vi "S4ACS.vi"() -> ()   [LabVIEW 2018]
uses:
  SPARC4_Channel/SPARC4_Channel.lvclass
  C:/Users/Denis/Desktop/S4ACS/S4ACS/Channel/Channel.lvclass
  Channel/Channel.lvclass/Channel.ctl
  Server/Server.lvclass/Server.ctl
  SPARC4_Channel/SPARC4_Channel.lvclass/SPARC4_Channel.ctl
  Sim_CCD/Sim_CCD.lvclass/Sim_CCD.ctl
  Sim_Ixon_Ultra/Sim_Ixon_Ultra.lvclass
  C:/Users/Denis/Desktop/S4ACS/S4ACS/Sim_CCD/Sim_CCD.lvclass
  <vilib>/Utility/error.llb/Error Cluster From Error Code.vi
  Sim_CCD/Sim_CCD.lvclass
  RxTx/RxTx.lvclass
  <vilib>/ErrorRing/Error Ring.xnode
  Channel/Channel.lvclass
  Server/Server.lvclass
panel:
  in  "generate error":bool
  out "error out":errorcluster
  in  "Tab Control":T1(tab)
  in  "Configuration to initialize ACS":T2={"image path"=path "C:/images/today", "channel"=1, "s4acs mode"=0, "log file path"=path "C:/sparc4/log/s4acs1", "min. log level"=0} {"min. log level" items=["STATUS", "DEBBUG", "INFO", "WARNING", "ERROR", "CRITICAL"]; "s4acs mode" items=["simulated", "real"]; "channel" min=1 max=4}
  out "S4GUI":bool
  out "S4ICS":bool
  out "TCS":bool
  out "Weather Station":bool
  out "Tel. focuser":bool
  out "wait expose cmd":bool
  in  "Stop Button":bool
  in  "software version":string="v1.56.0"
  out "ccd on/off":bool
  in  "use config file":bool=TRUE
  out "execution error":bool
  out "Numeric 2":i32
  out "Error Message":string
  out "Acquiring 2":bool
  out "Numeric":i32
  out "Code error message":string
  out "#cycles":u32
  out "cycles done":u16
  out "#seqs":u32
  out "seqs done":u16
  out "last update":string
  out "s4gui message":string
  out "last image":string
  out "frames done":u16
  out "ccd status":string
  out "temp (ºC)":i16
  out "temperature status":string
  out "exptime (s)":dbl
  out "serial number":u16
  out "Acquiring":bool
  out "#frames":u32
  in  "video mode":bool
  in  "reset axis":bool
  in  "contrast":dbl(slide)=1.0 scale=0.0..1.0
  in  "counts level":dbl(slide)=15.0 scale=0.0..5.0
  out "Intensity Graph":u16[][](graph)
  out "Header CCD Config":T3={"EM_GAIN"=2, "FRAME_TRANSFER"=TRUE, "SHUTTER_OPENING_TIME"=50, "SHUTTER_CLOSING_TIME"=50, "VBIN"=1, "INITIAL_LINE"=1, "INITIAL_COLUMN"=1, "FINAL_LINE"=1024, "FINAL_COLUMN"=1024, "HBIN"=1, "AD_CHANNEL"=0, "EM_MODE"=1, "PREAMP"=0, "SHUTTER_TTL"=0, "SHUTTER_MODE"=2, "ACQUISITION_MODE"=3, "TRIGGER_MODE"=0, "VERTICAL_CLOCK_VOLTAGE"=0, "VERTICAL_SHIFT_SPEED"=3, "READ_MODE"=4, "Last update"=timestamp(0 s since 1904-01-01), "READOUT_RATE"=""} {"READ_MODE" items=["Full Vertical Binning", "Multi-track", "Random-track", "Single-track", "Image"]; "VERTICAL_SHIFT_SPEED" items=["0.6", "1.13", "2.2", "4.33"]; "VERTICAL_CLOCK_VOLTAGE" items=["0", "+1", "+2", "+3", "+4"]; "TRIGGER_MODE" items=["Internal", "External", "N/A", "N/A_1", "N/A_2", "N/A_3", "External Start"]; "ACQUISITION_MODE" items=["Reserved", "Single", "Accumulate", "Kinetic"]; "SHUTTER_MODE" items=["Auto", "Open", "Closed"]; "SHUTTER_TTL" items=["TTL Low", "TTL High"]; "PREAMP" items=["Gain 1", "Gain 2"]; "EM_MODE" items=["Electron Multiplying", "Conventional"]}
  out "ACS status":string
  out "S4GUI":string
  out "S4ICS":string
  out "TCS":string
  out "Focuser":string
  out "Weather station":string
  out "SET erros":errorcluster
  out "Execution errors":errorcluster
  out "WRITE SETUP errors":errorcluster[](array[cluster])
  # "SPARC4 Acquisiton Control System (S4ACS)"
  # "Init communication"
  # "CCD status"
  # "ccd op. mode error"
  # "execution error"
  # "x1000"
  # "Camera configuration"
  # "Communication with the sub-systems of the observatory"
  # "Errors found during the exection of S4ACS"
  # "- Errors related to the WRITE SETUP command:"
  # "- Errors related to the SET command:"
  # "- Execution errors:"
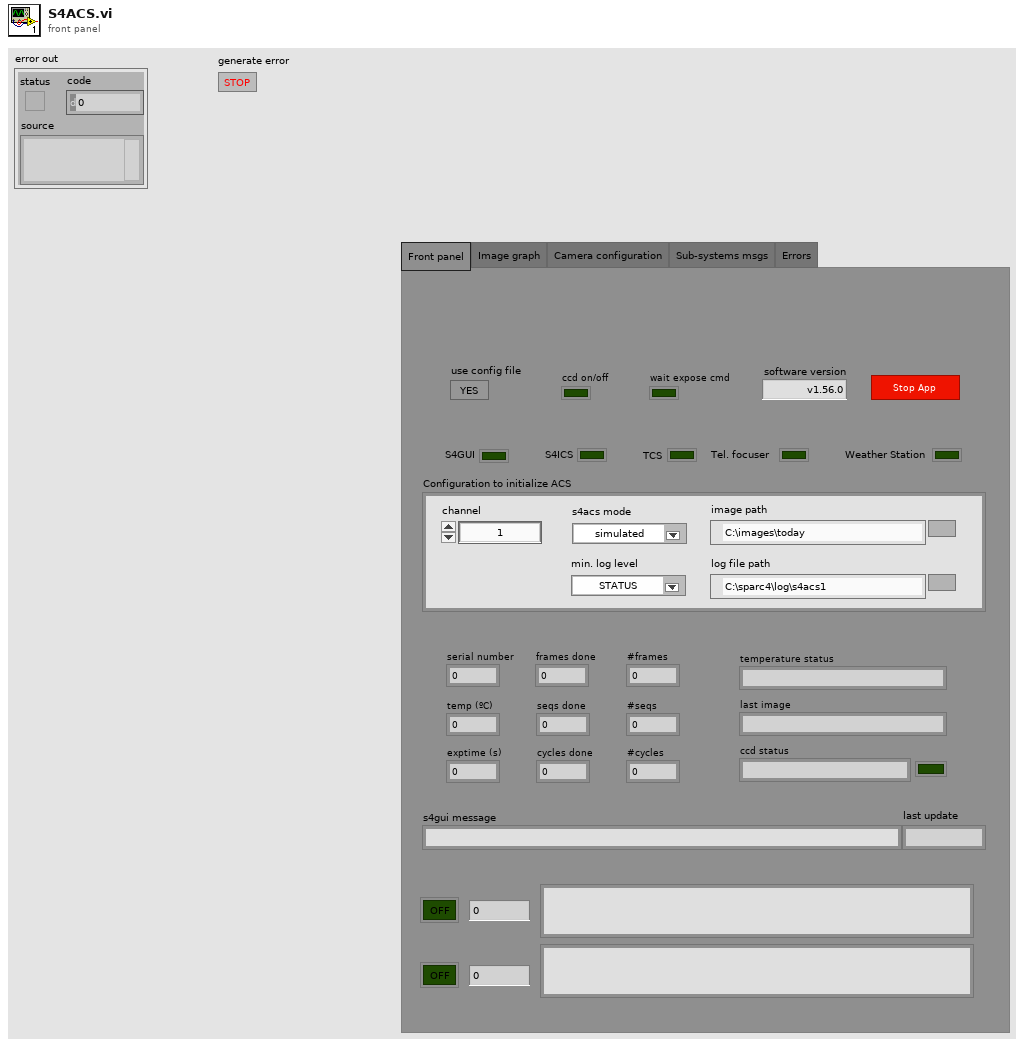
[diagram p1: front panel]
types:
  T1 = enum32{"Front panel", "Image graph", "Camera configuration", "Sub-systems msgs", "Errors"}
  T2 = cluster{"image path":path, "channel":u8, "s4acs mode":u16, "log file path":path, "min. log level":u16}
  T3 = cluster{"EM_GAIN":u16, "FRAME_TRANSFER":bool, "SHUTTER_OPENING_TIME":u16, "SHUTTER_CLOSING_TIME":u16, "VBIN":u16, "INITIAL_LINE":u16, "INITIAL_COLUMN":u16, "FINAL_LINE":u16, "FINAL_COLUMN":u16, "HBIN":u16, "AD_CHANNEL":u16, "EM_MODE":u16, "PREAMP":u16, "SHUTTER_TTL":u16, "SHUTTER_MODE":u16, "ACQUISITION_MODE":u16, "TRIGGER_MODE":u16, "VERTICAL_CLOCK_VOLTAGE":u16, "VERTICAL_SHIFT_SPEED":u16, "READ_MODE":u16, "Last update":timestamp, "READOUT_RATE":string}
  T4 = enum8{"Enabled", "Disabled", "Disabled and Grayed Out"}
  T5 = cluster{"Image path":path, "Channel":u8, "S4ACS mode":u16, "Log file path":path, "log level":u16}
  T6 = cluster{"Stop Acquisition":bool, "Abort Acquisition":bool, "Pause acquisition":bool, "wait expose command":bool, "video mode":bool, "stop app":bool}
  T7 = cluster{"State Machine.lvclass":refnum<class "State Machine.lvclass">, "RxTx.lvclass":refnum<class "RxTx.lvclass">, "Save_Header_RxTx.lvclass":refnum<class "RxTx.lvclass">, "Status SM.lvclass":refnum<class "State Machine.lvclass">, "Status RxTx.lvclass":refnum<class "RxTx.lvclass">, "servers array":refnum<class "Server.lvclass">[], "Events log file.lvclass":refnum<class "Log File.lvclass">, "Errors log file.lvclass":refnum<class "Log File.lvclass">, "Keywords log file.lvclass":refnum<class "Log File.lvclass">, "Sim_CCD.lvclass":refnum<class "Sim_CCD.lvclass">}
  T8 = cluster{"#SEQS":u32, "WAVEPLATE_POS":i32, "Waveplate positions":u8[]}
  T9 = cluster{"CYCLES_DONE":u16, "LAST_IMAGE_NAME":string, "USED_DISK_SPACE":u16, "IMAGE_INDEX":u32, "acquisition error":bool}
  T10 = cluster{"SEQS_DONE":u16, "S4ICS comm attempts":u8}
  T11 = cluster{"FRAMES_DONE":u16, "CCD_STATUS":string, "CURRENT_TEMPERATURE":i16, "TEMPERATURE_STATUS":string, "FRAME_EXPOSURE_TIME":sgl, "SERIAL_NUMBER":u16, "ACQUIRING":bool, "POWER":bool}
  T12 = cluster{"PREAMP":u16, "READOUT_RATE":u16, "VERTICAL_SHIFT_SPEED":u16, "READ_MODE":u16, "VERTICAL_CLOCK_VOLTAGE":u16, "ACQUISITION_MODE":u16, "AD_CHANNEL":u16, "SHUTTER_TTL":u16, "SHUTTER_OPENING_TIME":u16, "SHUTTER_CLOSING_TIME":u16, "SHUTTER_MODE":u16, "TRIGGER_MODE":u16, "VBIN":u16, "INITIAL_LINE":u16, "INITIAL_COLUMN":u16, "FINAL_LINE":u16, "FINAL_COLUMN":u16, "HBIN":u16, "TEMP":i32, "COOLER_POWER_STATUS":u16}
  T13 = cluster{"EM_MODE":u16, "EM_GAIN":u16, "FRAME_TRANSFER":bool}
  T14 = typedef "LVDateTimeRec.ctl" = cluster{"fractional second":dbl, "second":i32, "minute":i32, "hour":i32, "day of month":i32, "month":i32, "year":i32, "day of week":i32, "day of year":i32, "DST":i32}
  T15 = cluster{"Time Acq Started":u32, "Image delay":u64, "Last update - CCD config":timestamp, "SYSTEMTIME":T14, "Readout time":dbl, "Time acq finished":u32, "effective exptime":dbl}
  T16 = cluster{"CCD status":string, "camera op mode":string, "acq config":string, "GUI status msg":string, "op mode errors":string, "acq config error":string, "comm status":string}
  T17 = cluster{"#CYCLES":errorcluster, "SUFFIX":errorcluster}
  T18 = cluster{"#SEQS":errorcluster, "WAVEPLATE_POS":errorcluster}
  T19 = cluster{"EXPTIME":errorcluster, "#FRAMES":errorcluster}
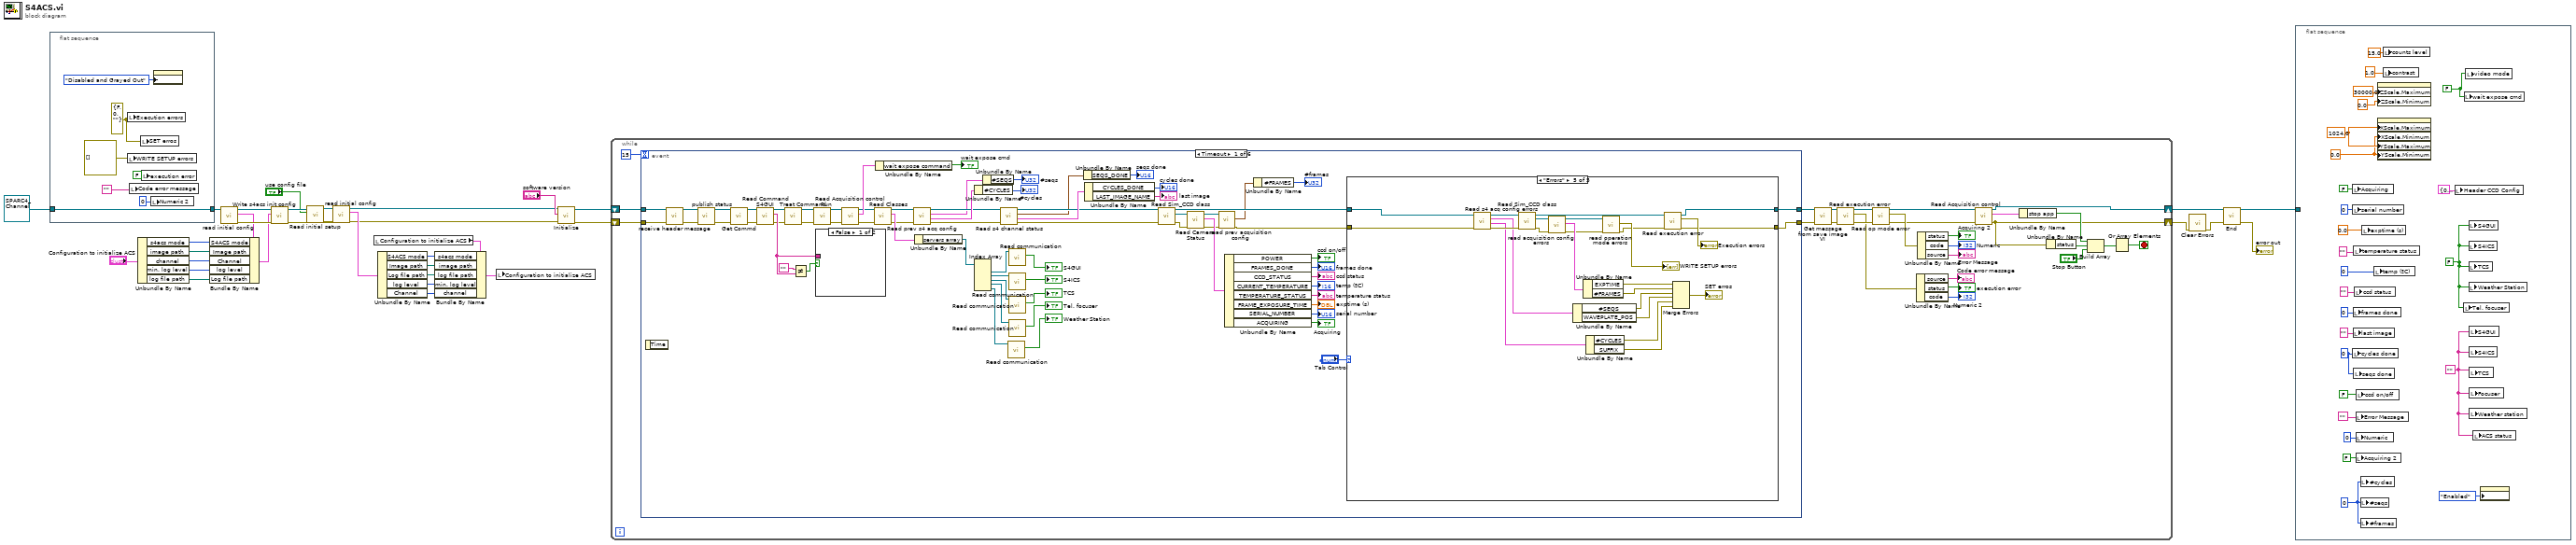
[diagram p0: block diagram]
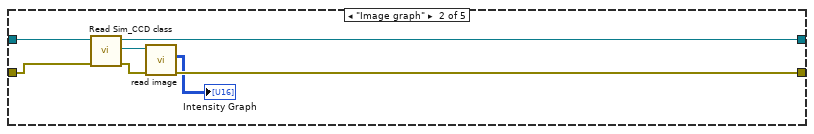
[diagram p3: hidden frame]
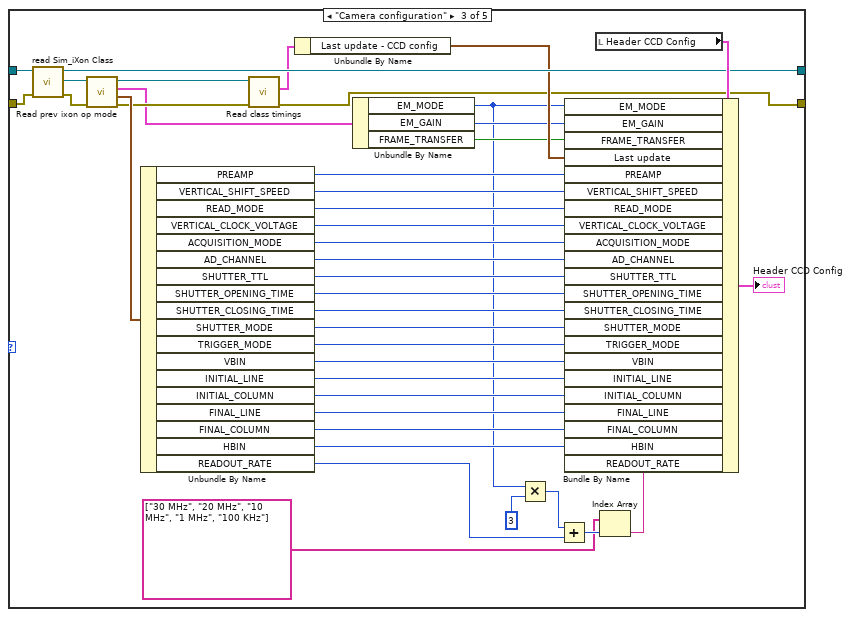
[diagram p4: hidden frame]
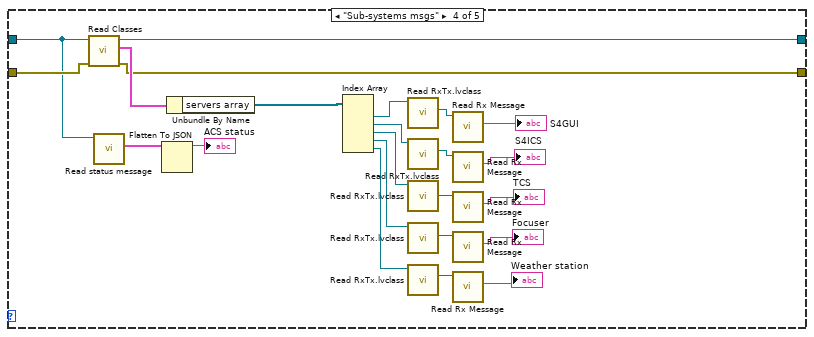
[diagram p5: hidden frame]
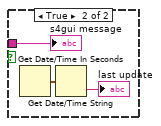
[diagram p6: hidden frame]
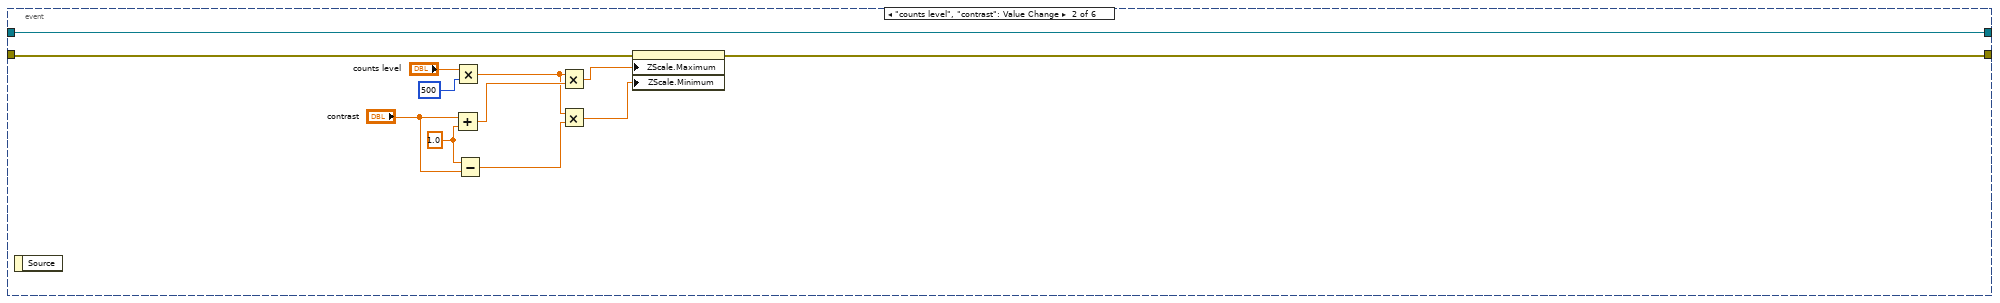
[diagram p7: hidden frame]
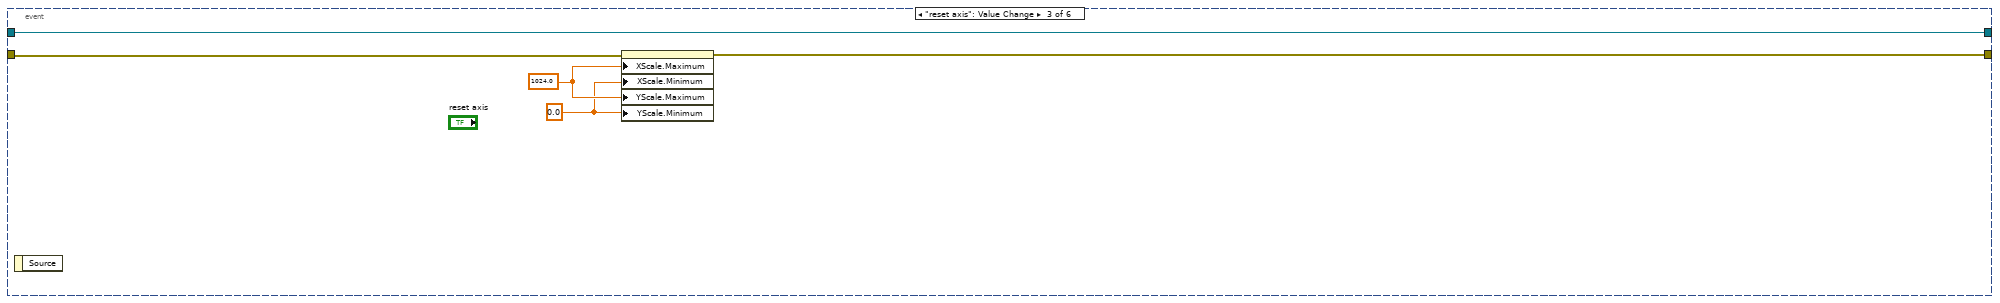
[diagram p8: hidden frame]
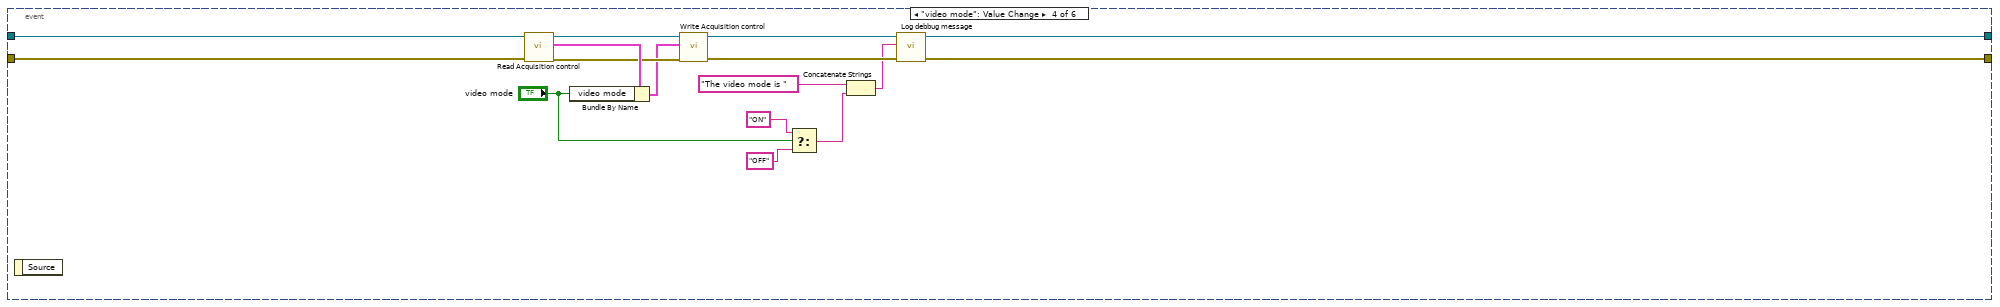
[diagram p9: hidden frame]
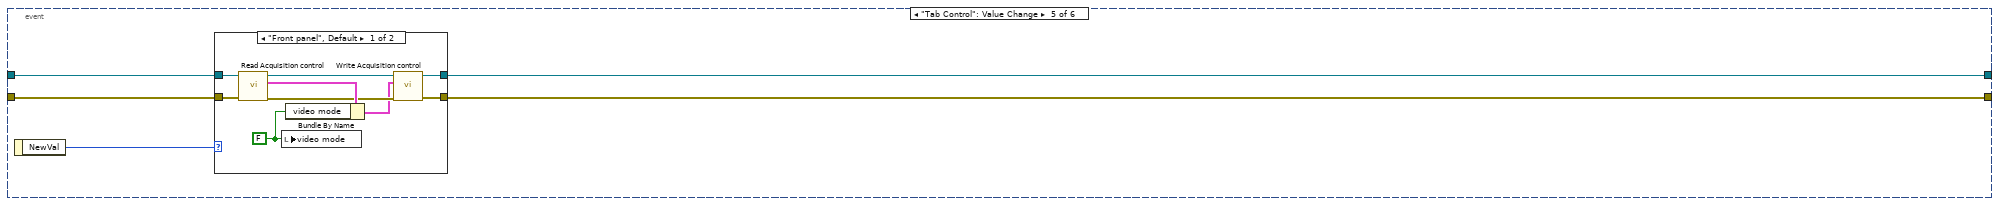
[diagram p10: hidden frame]
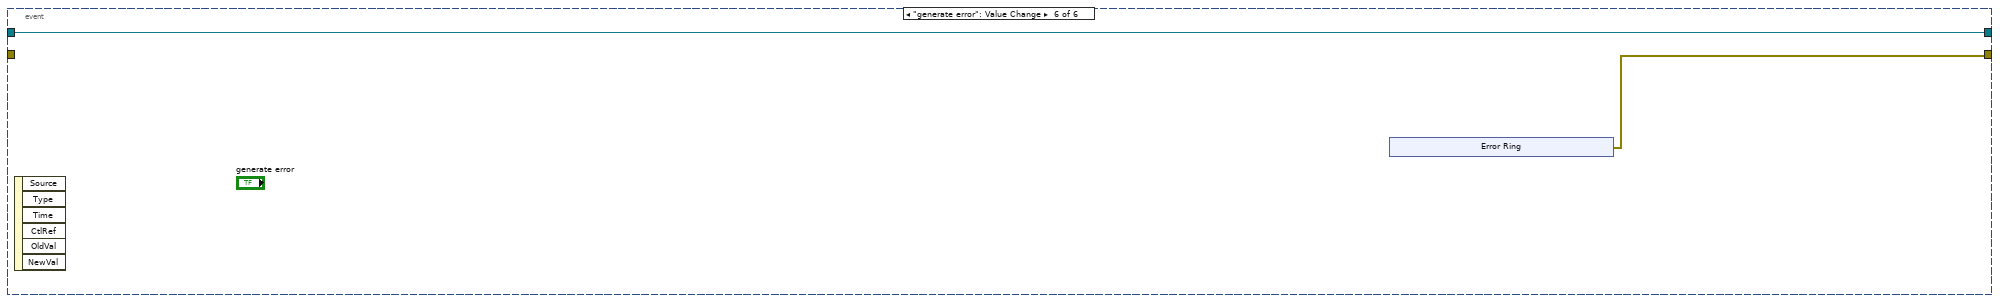
[diagram p12: hidden frame]
diagram:
  n1 = flat-sequence {
    tunnel: refnum<class "SPARC4_Channel.lvclass"> refnum ("SPARC4_Channel.lvclass") -> [w42]
    tunnel: [w42] -> w28
    frame #0 {
      w37 = errorcluster {"status"=FALSE, "code"=0, "source"=""} ("Execution errors")
      n2 = local write "Execution errors"(w37) -> ()
      n3 = local write "WRITE SETUP errors"(errorcluster[] [] ("WRITE SETUP errors")) -> ()
      n4 = local write "Code error message"("") -> ()
      n5 = local write "SET erros"(w37) -> ()
      n6 = local write "execution error"(FALSE ("Acquiring 3")) -> ()
      n7 = local write "Numeric 2"(0 ("Numeric 2")) -> ()
      n8 = property on="Configuration to initialize ACS" class="Clust (strict)"("DisabledEnum"=T4."Disabled and Grayed Out" ("Disabled")) -> ()  [unwired: 2 in, 2 out]
    }
  }
  n9 = Unbundle By Name("Configuration to initialize ACS") -> ("s4acs mode"=w22:u16, "image path"=w21:path, "channel"=w20:u8, "min. log level"=w19:u16, "log file path"=w17:path)
  n10 = call-dynamic "read initial config.vi"("Channel in"=w28) -> ("error out"=w26:errorcluster, "Configuration to initialize ACS"=w25:T5, "Channel out"=w27:refnum<class "SPARC4_Channel.lvclass">)  [unwired: 8 in]
  n11 = Bundle By Name(cluster=w25, "S4ACS mode"=w22, "Image path"=w21, "Channel"=w20, "log level"=w19, "Log file path"=w17) -> (w24:T5)
  n12 = call-dynamic "Write s4acs init config.vi"("error in (no error)"=w26, "Configuration to initialize ACS"=w24, "Channel in"=w27) -> ("error out"=w29:errorcluster, "Channel out"=w30:refnum<class "SPARC4_Channel.lvclass">)  [unwired: 7 in]
  n13 = call "Read initial setup.vi"("error in (no error)"=w29, "use cong file"="use config file", "Channel in"=w30) -> ("error out"=w7:errorcluster, "Channel out"=w8:refnum<class "SPARC4_Channel.lvclass">)  [unwired: 7 in]
  n14 = call-dynamic "read initial config.vi"("error in (no error)"=w7, "Channel in"=w8) -> ("error out"=w6:errorcluster, "Configuration to initialize ACS"=w9:T5, "Channel out"=w5:refnum<class "SPARC4_Channel.lvclass">)  [unwired: 7 in]
  n15 = local read "Configuration to initialize ACS"() -> (w11:T2)
  n16 = Unbundle By Name(w9) -> ("S4ACS mode"=w15:u16, "Image path"=w14:path, "Log file path"=w13:path, "log level"=w12:u16, "Channel"=w16:u8)
  n17 = Bundle By Name(cluster=w11, "s4acs mode"=w15, "image path"=w14, "log file path"=w13, "min. log level"=w12, "channel"=w16) -> (w10:T2)
  n18 = local write "Configuration to initialize ACS"(w10) -> ()
  n19 = call "Initialize.vi"("error IO"=w6, "Software version"="software version", "Channel.lvclass"=w5) -> ("error IO 2"=w35:errorcluster, "Channel.lvclass 2"=w34:refnum<class "SPARC4_Channel.lvclass">)  [unwired: 7 in]
  n20 = while {
    shift-right: [w45] -> w3
    shift-left: w35 -> [w68]
    shift-right: [w44] -> w33
    shift-left: w34 -> [w69]
    stop <- w54 stop-if-true
    n21 = event shown="[0] Timeout" {
      selector: _ -> [_ _ _ _ _ _]
      dyn-events: _ -> [_ _ _ _ _ _]
      timeout: 15 -> [_ _ _ _ _ _]
      tunnel: [w120 w246 w251 w260 w271 w286] -> w58
      tunnel: [w91 w248 w253 w261 w270 w287] -> w59
      tunnel: w69 -> [w117 w248 w253 w266 w273 w287]
      tunnel: w68 -> [w116 w247 w252 w265 w272 _]
      event Timeout {
        n22 = event-data() -> ()  [unwired: 1 in, 1 out]
        n23 = call "receive header message.vi"("error in (no error)"=w116, "Channel in"=w117) -> ("error out"=w115:errorcluster, "Channel out"=w114:refnum<class "SPARC4_Channel.lvclass">)  [unwired: 8 in]
        n24 = call "publish status.vi"("error in (no error)"=w115, "Channel in"=w114) -> ("error out"=w118:errorcluster, "Channel out"=w119:refnum<class "SPARC4_Channel.lvclass">)  [unwired: 8 in]
        n25 = call "Get Commd.vi"("error in (no error)"=w118, "Channel in"=w119) -> ("error out"=w123:errorcluster, "Channel out"=w124:refnum<class "SPARC4_Channel.lvclass">)  [unwired: 8 in]
        n26 = call "Read Command S4GUI.vi"("error in (no error)"=w123, "Channel in"=w124) -> ("error out"=w106:errorcluster, "Message"=w136:string, "Channel out"=w107:refnum<class "SPARC4_Channel.lvclass">)  [unwired: 7 in]
        n27 = call-dynamic "Treat Command.vi"("error in (no error)"=w106, "Channel in"=w107) -> ("error out"=w109:errorcluster, "Channel out"=w108:refnum<class "SPARC4_Channel.lvclass">)  [unwired: 8 in]
        n28 = Not Equal?(x="", y=w136) -> (x != y?=w137:bool)
        n29 = call-dynamic "Run.vi"("error in (no error)"=w109, "Channel in"=w108) -> ("error out"=w134:errorcluster, "Channel out"=w133:refnum<class "SPARC4_Channel.lvclass">)  [unwired: 8 in]
        n30 = case shown="False" w137 {
          tunnel: w136 -> [_ w236]
          frame False {
          }
          frame True {
            n31 = Get Date/Time In Seconds() -> (seconds since 1Jan1904=w235:timestamp)
            n32 = Get Date/Time String(seconds (now)=w235) -> (time string=→"last update":string)  [unwired: 2 in, 1 out]
            "s4gui message" <- w236
          }
        }
        n33 = call "Read Acquisition control.vi"("error in (no error)"=w134, "Channel in"=w133) -> ("error out"=w105:errorcluster, "Acquisition control"=w113:T6, "Channel out"=w104:refnum<class "SPARC4_Channel.lvclass">)  [unwired: 7 in]
        n34 = call-dynamic "Read Classes.vi"("error in (no error)"=w105, "Channel in"=w104) -> ("error out"=w89:errorcluster, "Classes"=w103:T7, "Channel out"=w88:refnum<class "SPARC4_Channel.lvclass">)  [unwired: 7 in]
        n35 = Unbundle By Name(w113) -> ("wait expose command"=→"wait expose cmd":bool)
        n36 = call "Read prev s4 acq config.vi"("error in (no error)"=w89, "SPARC4_Channel in"=w88) -> ("error out"=w81:errorcluster, "prev acq config"=w87:cluster{"suffix":string, "#CYCLES":u32}, "prev s4 acq config"=w73:T8, "SPARC4_Channel out"=w80:refnum<class "SPARC4_Channel.lvclass">)  [unwired: 6 in]
        n37 = Unbundle By Name(w103) -> ("servers array"=w90:refnum<class "Server.lvclass">[])
        n38 = Unbundle By Name(w87) -> ("#CYCLES"=→"#cycles":u32)
        n39 = Index Array(array=w90) -> (element #1=w102:refnum<class "Server.lvclass">, element #2=w101:refnum<class "Server.lvclass">, element #3=w100:refnum<class "Server.lvclass">, element #4=w99:refnum<class "Server.lvclass">, element #5=w98:refnum<class "Server.lvclass">)  [unwired: 5 in]
        n40 = Unbundle By Name(w73) -> ("#SEQS"=→"#seqs":u32)
        n41 = call "Read s4 channel status.vi"("error in (no error)"=w81, "SPARC4_Channel in"=w80) -> ("error out"=w78:errorcluster, "channel status"=w79:T9, "s4 channel status"=w71:T10, "SPARC4_Channel out"=w77:refnum<class "SPARC4_Channel.lvclass">)  [unwired: 6 in]
        n42 = call "Read communication.vi"("Server in"=w98) -> ("communication"=→"Weather Station":bool)  [unwired: 8 in, 2 out]
        n43 = call "Read communication.vi"("Server in"=w102) -> ("communication"=→"S4GUI":bool)  [unwired: 8 in, 2 out]
        n44 = call "Read communication.vi"("Server in"=w101) -> ("communication"=→"S4ICS":bool)  [unwired: 8 in, 2 out]
        n45 = call "Read communication.vi"("Server in"=w100) -> ("communication"=→"TCS":bool)  [unwired: 8 in, 2 out]
        n46 = call "Read communication.vi"("Server in"=w99) -> ("communication"=→"Tel. focuser":bool)  [unwired: 8 in, 2 out]
        n47 = Unbundle By Name(w71) -> ("SEQS_DONE"=→"seqs done":u16)
        n48 = Unbundle By Name(w79) -> ("CYCLES_DONE"=→"cycles done":u16, "LAST_IMAGE_NAME"=→"last image":string)
        n49 = call "Read Sim_CCD class.vi"("error in (no error)"=w78, "Channel in"=w77) -> ("error out"=w111:errorcluster, "Sim_CCD.lvclass"=w110:refnum<class "Sim_CCD.lvclass">, "Channel out"=w92:refnum<class "SPARC4_Channel.lvclass">)  [unwired: 7 in]
        n50 = call "Read Camera Status.vi"("error in (no error)"=w111, "CCDCamera in"=w110) -> ("error out"=w84:errorcluster, "camera status"=w132:T11, "CCDCamera out"=w85:refnum<class "Sim_CCD.lvclass">)  [unwired: 7 in]
        n51 = call "read prev acquisition config.vi"("error in (no error)"=w84, "Simulated_CCD_Camera in"=w85) -> ("error out"=w82:errorcluster, "Prev SET parameters"=w83:cluster{"EXPTIME":dbl, "#FRAMES":u32})  [unwired: 7 in, 1 out]
        n52 = Unbundle By Name(w132) -> ("POWER"=→"ccd on/off":bool, "FRAMES_DONE"=→"frames done":u16, "CCD_STATUS"=→"ccd status":string, "CURRENT_TEMPERATURE"=→"temp (ºC)":i16, "TEMPERATURE_STATUS"=→"temperature status":string, "FRAME_EXPOSURE_TIME"=→"exptime (s)":sgl, "SERIAL_NUMBER"=→"serial number":u16, "ACQUIRING"=→"Acquiring":bool)
        n53 = Unbundle By Name(w83) -> ("#FRAMES"=→"#frames":u32)
        n54 = case shown="\"Errors\"" "Tab Control" {
          tunnel: w82 -> [w139 w143 w159 w209 w216]
          tunnel: [w139 w146 w151 w207 w229] -> w120
          tunnel: w92 -> [w138 w144 w160 w187 w217]
          tunnel: [w138 w140 w156 w206 w230] -> w91
          frame "Front panel", Default {
          }
          frame "Image graph" {
            n55 = call "Read Sim_CCD class.vi"("error in (no error)"=w143, "Channel in"=w144) -> ("error out"=w142:errorcluster, "Sim_CCD.lvclass"=w141:refnum<class "Sim_CCD.lvclass">, "Channel out"=w140:refnum<class "SPARC4_Channel.lvclass">)  [unwired: 7 in]
            n56 = call "read image.vi"("error in (no error)"=w142, "CCDCamera in"=w141) -> ("error out"=w146:errorcluster, "Image Graph"=→"Intensity Graph":u16[][])  [unwired: 7 in, 1 out]
          }
          frame "Camera configuration" {
            n57 = call "read Sim_iXon Class.vi"("error in (no error)"=w159, "SPARC4_Channel in"=w160) -> ("error out"=w158:errorcluster, "Sim_Ixon_Ultra.lvclass"=w157:refnum<class "Sim_Ixon_Ultra.lvclass">, "SPARC4_Channel out"=w156:refnum<class "SPARC4_Channel.lvclass">)  [unwired: 7 in]
            n58 = call-dynamic "Read prev ixon op mode.vi"("error in (no error)"=w158, "Sim_Ixon_Ultra in"=w157) -> ("error out"=w155:errorcluster, "prev operation mode"=w186:T12, "prev ixon op mode"=w147:T13, "Sim_Ixon_Ultra out"=w154:refnum<class "Sim_Ixon_Ultra.lvclass">)  [unwired: 6 in]
            n59 = Unbundle By Name(w186) -> ("PREAMP"=w185:u16, "VERTICAL_SHIFT_SPEED"=w173:u16, "READ_MODE"=w172:u16, "VERTICAL_CLOCK_VOLTAGE"=w171:u16, "ACQUISITION_MODE"=w170:u16, "AD_CHANNEL"=w184:u16, "SHUTTER_TTL"=w169:u16, "SHUTTER_OPENING_TIME"=w183:u16, "SHUTTER_CLOSING_TIME"=w182:u16, "SHUTTER_MODE"=w168:u16, "TRIGGER_MODE"=w167:u16, "VBIN"=w181:u16, "INITIAL_LINE"=w180:u16, "INITIAL_COLUMN"=w179:u16, "FINAL_LINE"=w178:u16, "FINAL_COLUMN"=w177:u16, "HBIN"=w176:u16, "READOUT_RATE"=w164:u16)
            n60 = call "Read class timings.vi"("error in (no error)"=w155, "Simulated Camera in"=w154) -> ("error out"=w151:errorcluster, "class timings"=w153:T15)  [unwired: 7 in, 1 out]
            n61 = Unbundle By Name(w153) -> ("Last update - CCD config"=w152:timestamp)
            n62 = Unbundle By Name(w147) -> ("EM_MODE"=w148:u16, "EM_GAIN"=w150:u16, "FRAME_TRANSFER"=w149:bool)
            n63 = Multiply(x=w148, y=3) -> (x*y=w165:i32)
            n64 = Add(x=w165, y=w164) -> (x+y=w163:i32)
            n65 = local read "Header CCD Config"() -> (w174:T3)
            n66 = Index Array(array=string[] ["30 MHz", "20 MHz", "10 MHz", "1 MHz", "100 KHz"], index=w163) -> (element=w162:string)
            n67 = Bundle By Name(cluster=w174, "EM_MODE"=w148, "EM_GAIN"=w150, "FRAME_TRANSFER"=w149, "Last update"=w152, "PREAMP"=w185, "VERTICAL_SHIFT_SPEED"=w173, "READ_MODE"=w172, "VERTICAL_CLOCK_VOLTAGE"=w171, "ACQUISITION_MODE"=w170, "AD_CHANNEL"=w184, "SHUTTER_TTL"=w169, "SHUTTER_OPENING_TIME"=w183, "SHUTTER_CLOSING_TIME"=w182, "SHUTTER_MODE"=w168, "TRIGGER_MODE"=w167, "VBIN"=w181, "INITIAL_LINE"=w180, "INITIAL_COLUMN"=w179, "FINAL_LINE"=w178, "FINAL_COLUMN"=w177, "HBIN"=w176, "READOUT_RATE"=w162) -> (→"Header CCD Config":T3)
          }
          frame "Sub-systems msgs" {
            n68 = call-dynamic "Read Classes.vi"("error in (no error)"=w209, "Channel in"=w187) -> ("error out"=w207:errorcluster, "Classes"=w208:T7, "Channel out"=w206:refnum<class "SPARC4_Channel.lvclass">)  [unwired: 7 in]
            n69 = call "Read status message.vi"("Channel in"=w187) -> ("status message"=w188:T16)  [unwired: 8 in, 2 out]
            n70 = Flatten To JSON(anything=w188) -> (JSON string=→"ACS status":string)  [unwired: 2 in, 1 out]
            n71 = Unbundle By Name(w208) -> ("servers array"=w189:refnum<class "Server.lvclass">[])
            n72 = Index Array(array=w189) -> (element #1=w205:refnum<class "Server.lvclass">, element #2=w204:refnum<class "Server.lvclass">, element #3=w203:refnum<class "Server.lvclass">, element #4=w202:refnum<class "Server.lvclass">, element #5=w201:refnum<class "Server.lvclass">)  [unwired: 5 in]
            n73 = call "Read RxTx.lvclass.vi"("Server in"=w205) -> ("RxTx.lvclass"=w200:refnum<class "RxTx.lvclass">)  [unwired: 8 in, 2 out]
            n74 = call "Read RxTx.lvclass.vi"("Server in"=w204) -> ("RxTx.lvclass"=w199:refnum<class "RxTx.lvclass">)  [unwired: 8 in, 2 out]
            n75 = call "Read RxTx.lvclass.vi"("Server in"=w203) -> ("RxTx.lvclass"=w198:refnum<class "RxTx.lvclass">)  [unwired: 8 in, 2 out]
            n76 = call "Read RxTx.lvclass.vi"("Server in"=w202) -> ("RxTx.lvclass"=w197:refnum<class "RxTx.lvclass">)  [unwired: 8 in, 2 out]
            n77 = call "Read RxTx.lvclass.vi"("Server in"=w201) -> ("RxTx.lvclass"=w196:refnum<class "RxTx.lvclass">)  [unwired: 8 in, 2 out]
            n78 = call "Read Rx Message.vi"("RxTx in"=w200) -> ("Rx Message"=→"S4GUI":string)  [unwired: 8 in, 2 out]
            n79 = call "Read Rx Message.vi"("RxTx in"=w199) -> ("Rx Message"=→"S4ICS":string)  [unwired: 8 in, 2 out]
            n80 = call "Read Rx Message.vi"("RxTx in"=w198) -> ("Rx Message"=→"TCS":string)  [unwired: 8 in, 2 out]
            n81 = call "Read Rx Message.vi"("RxTx in"=w197) -> ("Rx Message"=→"Focuser":string)  [unwired: 8 in, 2 out]
            n82 = call "Read Rx Message.vi"("RxTx in"=w196) -> ("Rx Message"=→"Weather station":string)  [unwired: 8 in, 2 out]
          }
          frame "Errors" {
            n83 = call "Read s4 acq config errors.vi"("error in (no error)"=w216, "SPARC4_Channel in"=w217) -> ("error out"=w219:errorcluster, "acquisition config errors"=w212:T17, "s4 acq config errors"=w213:T18, "SPARC4_Channel out"=w218:refnum<class "SPARC4_Channel.lvclass">)  [unwired: 6 in]
            n84 = call "Read Sim_CCD class.vi"("error in (no error)"=w219, "Channel in"=w218) -> ("error out"=w220:errorcluster, "Sim_CCD.lvclass"=w224:refnum<class "Sim_CCD.lvclass">, "Channel out"=w232:refnum<class "SPARC4_Channel.lvclass">)  [unwired: 7 in]
            n85 = call "read acquisition config errors.vi"("error in (no error)"=w220, "Simulated Camera in"=w224) -> ("error out"=w221:errorcluster, "acq config errors"=w225:T19, "Simulated Camera out"=w222:refnum<class "Sim_CCD.lvclass">)  [unwired: 7 in]
            n86 = Unbundle By Name(w213) -> ("#SEQS"=w215:errorcluster, "WAVEPLATE_POS"=w214:errorcluster)
            n87 = Unbundle By Name(w225) -> ("EXPTIME"=w228:errorcluster, "#FRAMES"=w227:errorcluster)
            n88 = Unbundle By Name(w212) -> ("#CYCLES"=w211:errorcluster, "SUFFIX"=w210:errorcluster)
            n89 = call "read operation mode errors.vi"("error in (no error)"=w221, "Simulated_CCD_Camera in"=w222) -> ("error out"=w223:errorcluster, "WRITE SETUP errors"=→"WRITE SETUP errors":errorcluster[])  [unwired: 7 in, 1 out]
            n90 = call-dynamic "Read execution error.vi"("error in (no error)"=w223, "Channel in"=w232) -> ("error out"=w229:errorcluster, "execution error"=→"Execution errors":errorcluster, "Channel out"=w230:refnum<class "SPARC4_Channel.lvclass">)  [unwired: 7 in]
            n91 = Merge Errors(w228, w227, w215, w214, w211, w210) -> (→"SET erros":errorcluster)
          }
        }
      }
      event "counts level", "contrast": Value Change {
        w240 = 1.0
        n92 = event-data() -> ()  [unwired: 1 in, 1 out]
        n93 = Add(x="contrast", y=w240) -> (x+y=w243:dbl)
        n94 = Multiply(x="counts level", y=500) -> (x*y=w238:dbl)
        n95 = Subtract(x=w240, y="contrast") -> (x-y=w239:dbl)
        n96 = Multiply(x=w238, y=w243) -> (x*y=w242:dbl)
        n97 = Multiply(x=w238, y=w239) -> (x*y=w241:dbl)
        n98 = property on="Intensity Graph" class="IntGraph (strict)"(error in=w247, "ZScale.Maximum"=w242, "ZScale.Minimum"=w241) -> (error out=w246:errorcluster)  [unwired: 1 in, 1 out]
      }
      event "reset axis": Value Change {
        w249 = 0.0
        w250 = 1024.0
        n99 = event-data() -> ()  [unwired: 1 in, 1 out]
        n100 = property on="Intensity Graph" class="IntGraph (strict)"(error in=w252, "XScale.Maximum"=w250, "XScale.Minimum"=w249, "YScale.Maximum"=w250, "YScale.Minimum"=w249) -> (error out=w251:errorcluster)  [unwired: 1 in, 1 out]
      }
      event "video mode": Value Change {
        n101 = event-data() -> ()  [unwired: 1 in, 1 out]
        n102 = call "Read Acquisition control.vi"("error in (no error)"=w265, "Channel in"=w266) -> ("error out"=w268:errorcluster, "Acquisition control"=w269:T6, "Channel out"=w267:refnum<class "SPARC4_Channel.lvclass">)  [unwired: 7 in]
        n103 = Bundle By Name(cluster=w269, "video mode"="video mode") -> (w264:T6)
        n104 = call "Write Acquisition control.vi"("error in (no error)"=w268, "Acquisition control"=w264, "Channel in"=w267) -> ("error out"=w263:errorcluster, "Channel out"=w262:refnum<class "SPARC4_Channel.lvclass">)  [unwired: 7 in]
        n105 = Select(t="ON", s="video mode", f="OFF") -> (s? t:f=w257:string)
        n106 = Concatenate Strings("The video mode is ", w257) -> (w259:string)
        n107 = call "Log debbug message.vi"("error in (no error)"=w263, "String"=w259, "Channel in"=w262) -> ("error out"=w260:errorcluster, "Channel out"=w261:refnum<class "SPARC4_Channel.lvclass">)  [unwired: 7 in]
      }
      event "Tab Control": Value Change {
        n108 = event-data() -> ("NewVal"=w274:T1)  [unwired: 1 in]
        n109 = case shown="\"Front panel\", Default" w274 {
          tunnel: w273 -> [w282 w285]
          tunnel: w272 -> [w283 w284]
          tunnel: [w281 w284] -> w271
          tunnel: [w280 w285] -> w270
          frame "Front panel", Default {
            w278 = FALSE ("video mode")
            n110 = call "Read Acquisition control.vi"("error in (no error)"=w283, "Channel in"=w282) -> ("error out"=w277:errorcluster, "Acquisition control"=w279:T6, "Channel out"=w276:refnum<class "SPARC4_Channel.lvclass">)  [unwired: 7 in]
            n111 = local write "video mode"(w278) -> ()
            n112 = Bundle By Name(cluster=w279, "video mode"=w278) -> (w275:T6)
            n113 = call "Write Acquisition control.vi"("error in (no error)"=w277, "Acquisition control"=w275, "Channel in"=w276) -> ("error out"=w281:errorcluster, "Channel out"=w280:refnum<class "SPARC4_Channel.lvclass">)  [unwired: 7 in]
          }
          frame "Image graph" {
          }
        }
      }
      event "generate error": Value Change {
        n114 = event-data() -> ()  [unwired: 1 in, 6 out]
        n115 = xnode "Error Ring"() -> ("error out"=w286:errorcluster)
      }
    }
    n116 = call "Get message from save image VI.vi"("error in (no error)"=w58, "Channel in"=w59) -> ("error out"=w60:errorcluster, "Channel out"=w61:refnum<class "SPARC4_Channel.lvclass">)  [unwired: 8 in]
    n117 = call-dynamic "Read execution error.vi"("error in (no error)"=w60, "Channel in"=w61) -> ("error out"=w50:errorcluster, "execution error"=w43:errorcluster, "Channel out"=w62:refnum<class "SPARC4_Channel.lvclass">)  [unwired: 7 in]
    n118 = call-dynamic "Read op mode error.vi"("error in (no error)"=w50, "Channel in"=w62) -> ("error out"=w46:errorcluster, "system error"=w66:errorcluster, "Channel out"=w48:refnum<class "SPARC4_Channel.lvclass">)  [unwired: 7 in]
    n119 = Unbundle By Name(w43) -> ("source"=→"Code error message":string, "status"=→"execution error":bool, "code"=→"Numeric 2":i32)
    n120 = Unbundle By Name(w66) -> ("status"=→"Acquiring 2":bool, "code"=→"Numeric":i32, "source"=→"Error Message":string)
    n121 = call "Read Acquisition control.vi"("error in (no error)"=w46, "Channel in"=w48) -> ("error out"=w45:errorcluster, "Acquisition control"=w49:T6, "Channel out"=w44:refnum<class "SPARC4_Channel.lvclass">)  [unwired: 7 in]
    n122 = Unbundle By Name(w49) -> ("stop app"=w47:bool)
    n123 = Unbundle By Name(w45) -> ("status"=w57:bool)
    n124 = Build Array(w47, w57, "Stop Button") -> (w55:bool[])
    n125 = Or Array Elements(Boolean array=w55) -> (logical OR=w54:bool)
  }
  n126 = call <vilib>:"Clear Errors.vi"("error in (no error)"=w3) -> ("error out"=w2:errorcluster)  [unwired: 5 in, 1 out]
  n127 = call "End.vi"("error in (no error)"=w2, "Channel in"=w33) -> ("error out"=→"error out":errorcluster, "Channel out"=w32:refnum<class "SPARC4_Channel.lvclass">)  [unwired: 8 in]
  n128 = flat-sequence {
    tunnel: w32 -> [_]
    frame #0 {
      w293 = 0 ("Numeric")
      w295 = ""
      w299 = FALSE
      w301 = FALSE ("Acquiring")
      w307 = 0.0
      w308 = 1024.0
      w302 = u16 0 ("Cubes done")
      n129 = local write "Acquiring"(FALSE ("Acquiring")) -> ()
      n130 = local write "serial number"(u16 0 ("Serial number")) -> ()
      n131 = local write "cycles done"(w302) -> ()
      n132 = local write "frames done"(u16 0 ("Frames done")) -> ()
      n133 = local write "last image"("" ("Last image")) -> ()
      n134 = local write "temperature status"("" ("Temperature status")) -> ()
      n135 = local write "seqs done"(w302) -> ()
      n136 = local write "ccd status"("" ("CCD status")) -> ()
      n137 = local write "Error Message"("") -> ()
      n138 = local write "Numeric"(0 ("Numeric")) -> ()
      n139 = local write "Acquiring 2"(FALSE ("Acquiring 2")) -> ()
      n140 = local write "ccd on/off"(FALSE ("CCD ON/OFF")) -> ()
      n141 = local write "#cycles"(w293) -> ()
      n142 = local write "#seqs"(w293) -> ()
      n143 = local write "#frames"(w293) -> ()
      n144 = local write "exptime (s)"(0.0 ("Frame exptime (s)")) -> ()
      n145 = local write "temp (ºC)"(i16 0 ("Current temperature (ºC)")) -> ()
      n146 = property on="Intensity Graph" class="IntGraph (strict)"("ZScale.Maximum"=30000.0, "ZScale.Minimum"=0.0) -> ()  [unwired: 2 in, 2 out]
      n147 = property on="Intensity Graph" class="IntGraph (strict)"("XScale.Maximum"=w308, "XScale.Minimum"=w307, "YScale.Maximum"=w308, "YScale.Minimum"=w307) -> ()  [unwired: 2 in, 2 out]
      n148 = local write "counts level"(15.0) -> ()
      n149 = local write "contrast"(1.0) -> ()
      n150 = local write "Header CCD Config"(T3 {"EM_GAIN"=0, "FRAME_TRANSFER"=FALSE, "SHUTTER_OPENING_TIME"=0, "SHUTTER_CLOSING_TIME"=0, "VBIN"=0, "INITIAL_LINE"=0, "INITIAL_COLUMN"=0, "FINAL_LINE"=0, "FINAL_COLUMN"=0, "HBIN"=0, "AD_CHANNEL"=0, "EM_MODE"=1, "PREAMP"=0, "SHUTTER_TTL"=0, "SHUTTER_MODE"=2, "ACQUISITION_MODE"=3, "TRIGGER_MODE"=0, "VERTICAL_CLOCK_VOLTAGE"=0, "VERTICAL_SHIFT_SPEED"=3, "READ_MODE"=4, "Last update"=timestamp(0 s since 1904-01-01), "READOUT_RATE"=""} ("Header CCD Config")) -> ()
      n151 = local write "Tel. focuser"(w299) -> ()
      n152 = local write "wait expose cmd"(w301) -> ()
      n153 = local write "video mode"(w301) -> ()
      n154 = local write "S4GUI"(w299) -> ()
      n155 = local write "S4ICS"(w299) -> ()
      n156 = local write "TCS"(w299) -> ()
      n157 = local write "Weather Station"(w299) -> ()
      n158 = local write "S4GUI"(w295) -> ()
      n159 = local write "S4ICS"(w295) -> ()
      n160 = local write "TCS"(w295) -> ()
      n161 = local write "Focuser"(w295) -> ()
      n162 = local write "Weather station"(w295) -> ()
      n163 = local write "ACS status"(w295) -> ()
      n164 = property on="Configuration to initialize ACS" class="Clust (strict)"("DisabledEnum"=T4."Enabled" ("Disabled")) -> ()  [unwired: 2 in, 2 out]
    }
  }
